vi "列表框选择添加项目(dbclick).vi"() -> ()   [LabVIEW 2012, in "Listbox Tool.lvlib"]
uses:
  Listbox Tool.lvlib
  Method/Get Item From Index.vi
  Method/Add Item.vi
  Method/Delete Item By Index.vi
panel:
  in  "停止":bool
  in  "已选择动作":i32(listbox)
  in  "红绿灯动作":i32(listbox)=8
  # "双击添加"
  # "双击删除"
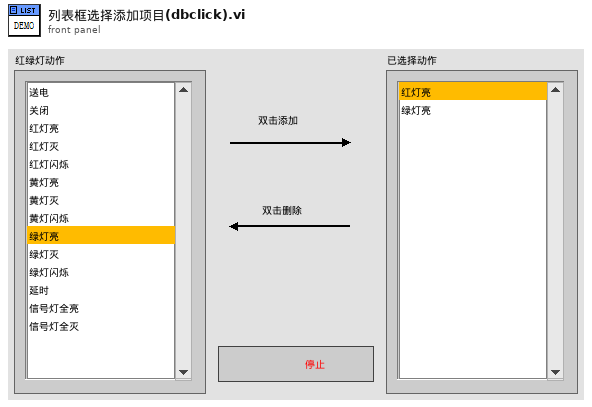
[diagram p1: front panel]
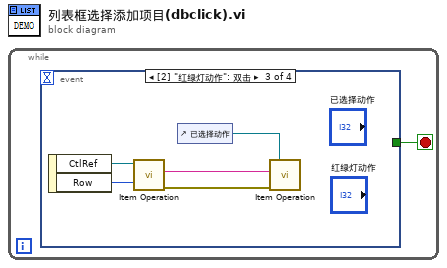
[diagram p0: block diagram]
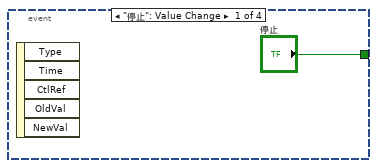
[diagram p2: hidden frame]
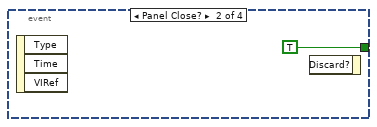
[diagram p3: hidden frame]
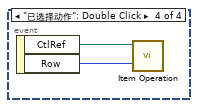
[diagram p4: hidden frame]
diagram:
  n1 = while {
    stop <- w1 stop-if-true
    n2 = event shown="[2] \"红绿灯动作\": 双击" {
      selector: _ -> [_ _ _ _]
      dyn-events: _ -> [_ _ _ _]
      timeout: _ -> [_ _ _ _]
      tunnel: ["停止" TRUE ("停止") _ _] -> w1
      event "停止": Value Change {
        n3 = event-data() -> ()  [unwired: 1 in, 5 out]
      }
      event Panel Close? {
        n4 = event-data() -> ()  [unwired: 1 in, 3 out]
        n5 = event-data() -> ()  [unwired: 2 in, 1 out]
      }
      event "红绿灯动作": Double Click {
        n6 = event-data() -> ("CtlRef"=w8:refnum<vi>, "Row"=w4:i32)  [unwired: 1 in]
        n7 = call-poly "Item Operation.vi"("Index"=w4, "Listbox Ref"=w8) -> ("错误输出"=w7:errorcluster, "Item"=w6:string)  [unwired: 7 in, 1 out]
        n8 = control-ref of="已选择动作"() -> (w5:refnum<vi>)
        n9 = call-poly "Item Operation.vi"("错误输入"=w7, "Item"=w6, "Listbox Ref"=w5) -> ()  [unwired: 7 in, 2 out]
      }
      event "已选择动作": Double Click {
        n10 = event-data() -> ("CtlRef"=w10:refnum<vi>, "Row"=w9:i32)  [unwired: 1 in]
        n11 = call-poly "Item Operation.vi"("Index"=w9, "Listbox Ref"=w10) -> ()  [unwired: 8 in, 2 out]
      }
    }
  }
